vi "Splitting_filename.vi"(10 "Splitting number":u32, 11 "Total filenames":string[](array[string])) -> (3 "Splitted filenames":string[][](array[string]))   [LabVIEW 2021]
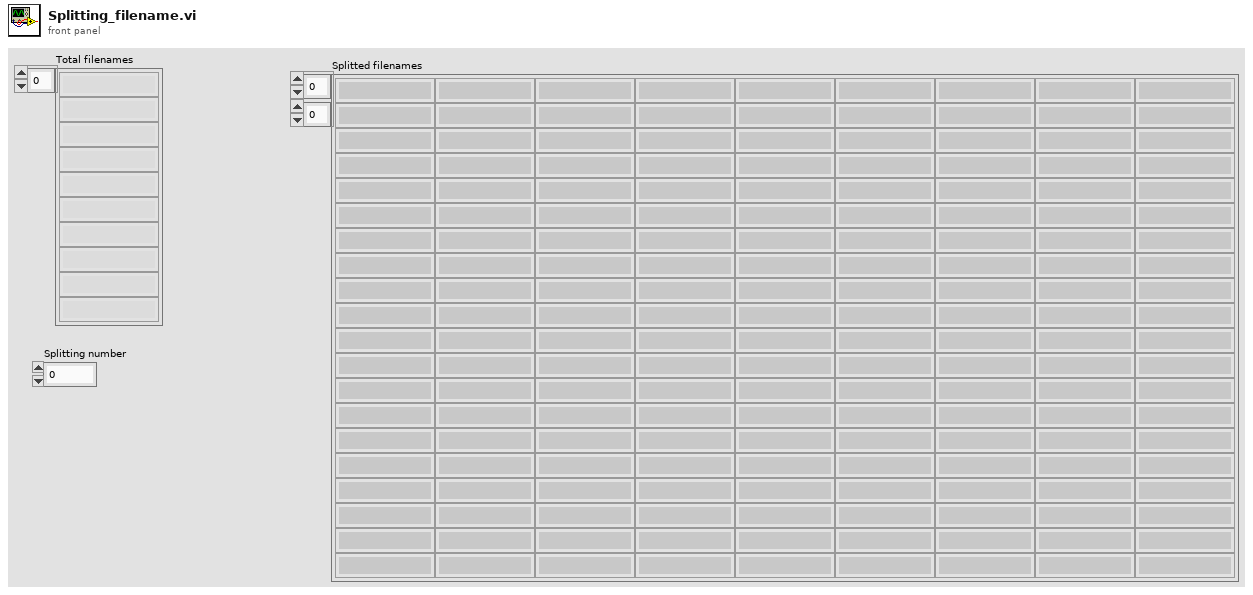
[diagram p1: front panel]
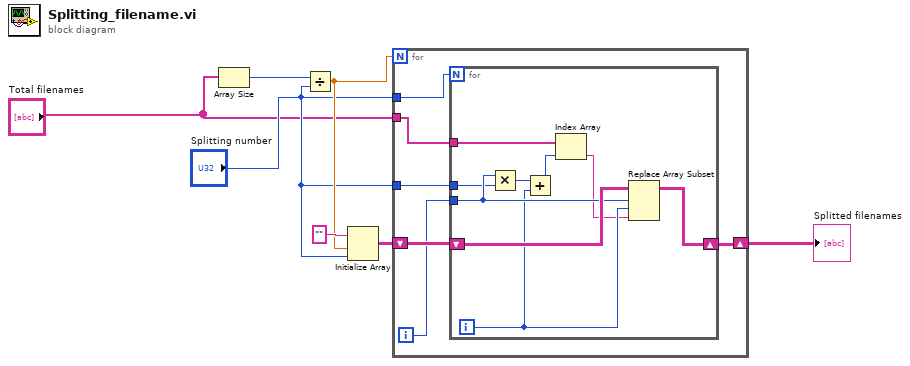
[diagram p0: block diagram]
diagram:
  n1 = Array Size(array="Total filenames") -> (size(s)=w7:i32)
  n2 = Divide(x=w7, y="Splitting number") -> (x/y=w4:dbl)
  n3 = Initialize Array("", w4, "Splitting number") -> (w5:string[][])
  n4 = for {
    N: w4 -> [_]
    tunnel: "Total filenames" -> [w12]
    shift-right: [w10] -> w2
    shift-left: w5 -> [w13]
    tunnel: "Splitting number" -> [w9]
    tunnel: "Splitting number" -> [w8]
    i -> [w11]
    n5 = for {
      N: w9 -> [_]
      tunnel: w12 -> [w20]
      shift-right: [w21] -> w10
      shift-left: w13 -> [w22]
      tunnel: w11 -> [w19]
      tunnel: w8 -> [w14]
      i -> [w17]
      n6 = Multiply(x=w19, y=w14) -> (x*y=w18:u32)
      n7 = Add(x=w18, y=w17) -> (x+y=w16:u32)
      n8 = Index Array(array=w20, index=w16) -> (element=w15:string)
      n9 = Replace Array Subset(array=w22, new element=w15, index (row)=w19, index (col)=w17) -> (w21:string[][])
    }
  }
  "Splitted filenames" <- w2
